vi "2 - Event vs Queue Benchmark.vi"() -> ()   [LabVIEW 2012]
uses:
  <vilib>/picture/picture.llb/imagedata.ctl
panel:
  out "Queue 2":cluster{u32, u32, u32}[](array[cluster])=[{8, 476, 0}, {8, 479, 0}, {6, 476, 0}, {7, 480, 0}, {8, 553, 0}, {8, 483, 0}, {8, 475, 0}, {9, 578, 0}, {10, 578, 0}, {8, 478, 0}, {9, 503, 0}, {9, 573, 0}, {8, 530, 0}, {8, 476, 0}, {8, 478, 0}, {8, 480, 0}, {8, 501, 0}, {7, 481, 0}, {7, 499, 0}, {7, 480, 0}]
  out "Event":cluster{u32, u32, u32}[](array[cluster])=[{24, 585, 0}, {22, 555, 0}, {21, 500, 0}, {23, 505, 0}, {25, 507, 0}, {24, 517, 0}, {20, 506, 0}, {23, 505, 0}, {23, 570, 0}, {23, 503, 0}, {23, 523, 0}, {23, 589, 0}, {25, 701, 0}, {24, 716, 0}, {25, 675, 1}, {24, 650, 0}, {22, 585, 0}, {25, 612, 0}, {22, 502, 0}, {23, 499, 0}]
  out "Time to Create":u32
  out "Time to Enqueue":u32
  out "Time to Handle":u32
  out "MB Buffered":dbl
  out "Picture 1":picture
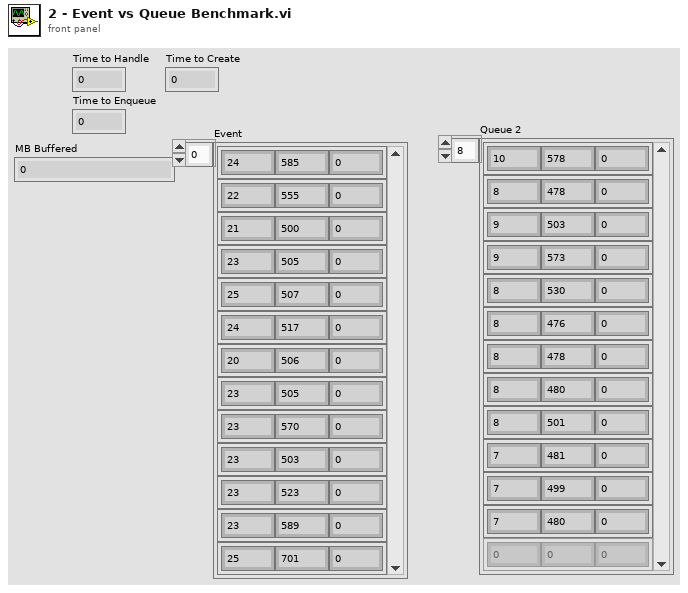
[diagram p1: front panel]
types:
  T1 = typedef "imagedata.ctl" = cluster{"image type":i32, "image depth":i32, "image":u8[], "mask":u8[], "colors":u32[], "Rectangle":cluster{"left":i16, "top":i16, "right":i16, "bottom":i16}}
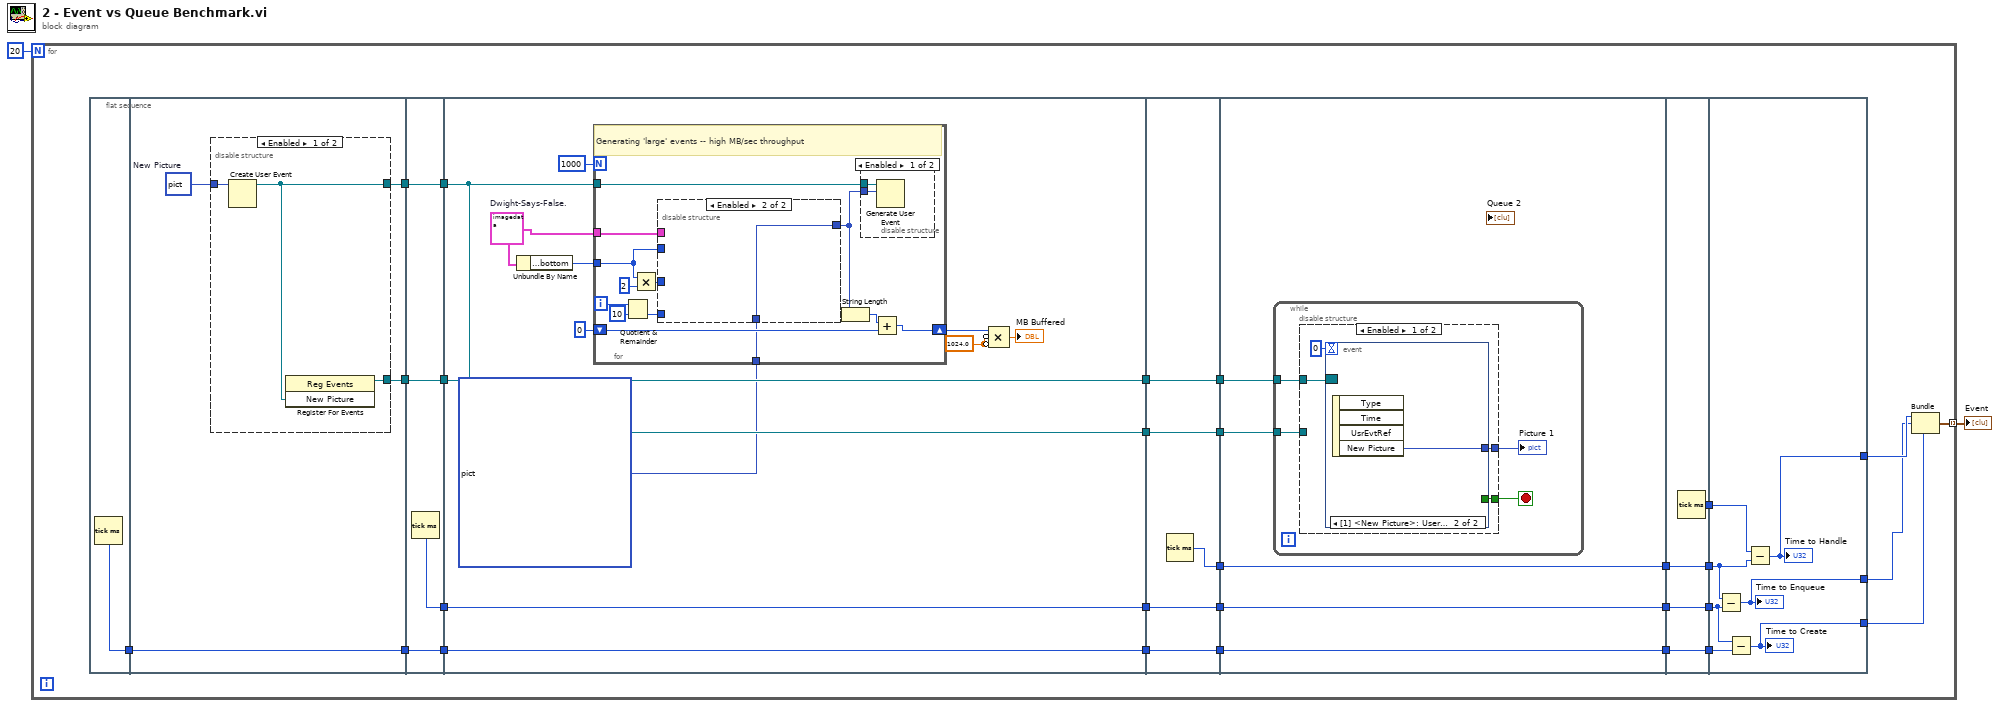
[diagram p0: block diagram]
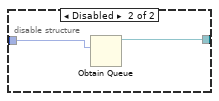
[diagram p2: hidden frame]
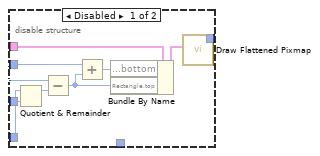
[diagram p3: hidden frame]
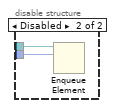
[diagram p4: hidden frame]
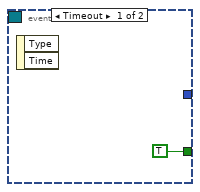
[diagram p5: hidden frame]
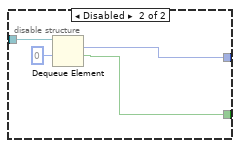
[diagram p6: hidden frame]
diagram:
  n1 = for {
    N: 20 -> [_]
    tunnel: [w3] -> w1 mode=indexing
    n2 = flat-sequence {
      tunnel: [w31] -> w30
      tunnel: [w35] -> w29
      tunnel: [w34] -> w28
      tunnel: w30 -> [w32]
      tunnel: [w32] -> w27
      tunnel: w29 -> [w44]
      tunnel: [w44] -> w26
      tunnel: w28 -> [w43]
      tunnel: [w43] -> w25
      tunnel: [w42] -> w24
      tunnel: w27 -> [w41]
      tunnel: [w41] -> w23
      tunnel: w26 -> [w49]
      tunnel: w25 -> [w50]
      tunnel: [w50] -> w22
      tunnel: [w49] -> w21
      tunnel: w24 -> [w48]
      tunnel: [w48] -> w20
      tunnel: w23 -> [w47]
      tunnel: [w47] -> w19
      tunnel: w22 -> [w88]
      tunnel: [w88] -> w18
      tunnel: [w87] -> w17
      tunnel: w21 -> [w87]
      tunnel: [w86] -> w16
      tunnel: w20 -> [w85]
      tunnel: [w85] -> w15
      tunnel: w19 -> [w84]
      tunnel: [w84] -> w14
      tunnel: w18 -> [w93]
      tunnel: w17 -> [w92]
      tunnel: [w91] -> w13
      tunnel: w16 -> [w91]
      tunnel: w15 -> [w90]
      tunnel: [w90] -> w12
      tunnel: w14 -> [w89]
      tunnel: [w89] -> w11
      tunnel: [w111] -> w10
      tunnel: [w110] -> w9
      tunnel: w13 -> [w110]
      tunnel: w12 -> [w109]
      tunnel: [w109] -> w8
      tunnel: w11 -> [w108]
      tunnel: [w108] -> w7
      tunnel: w10 -> [w118]
      tunnel: w9 -> [w117]
      tunnel: w8 -> [w116]
      tunnel: w7 -> [w115]
      tunnel: [w114] -> w6
      tunnel: [w113] -> w5
      tunnel: [w112] -> w4
      frame #0 {
        n3 = Tick Count (ms)() -> (millisecond timer value=w31:u32)
      }
      frame #1 {
        w33 = picture data[5B]  # New Picture
        n4 = disable-structure shown="Enabled" {
          disable-tunnel: [w38 w39] -> w35
          disable-tunnel: [w37 _] -> w34
          disable-tunnel: w33 -> [w36 w40]
          frame Enabled {
            n5 = Create User Event(user event datatype=w36) -> (user event=w38:refnum<user-event>)  [unwired: 1 in, 1 out]
            n6 = register-events(w38) -> (reference out=w37:refnum<event-registration>)  [unwired: 2 in, 1 out]
          }
          frame Disabled {
            n7 = Obtain Queue(element data type=w40) -> (queue out=w39:refnum<queue>)  [unwired: 4 in, 2 out]
          }
        }
      }
      frame #2 {
        n8 = Tick Count (ms)() -> (millisecond timer value=w42:u32)
      }
      frame #3 {
        w54 = 1024.0 ("value")
        w46 = T1 {"image type"=0, "image depth"=32, "image"=array[234768 elements], "mask"=array[7504 elements], "colors"=[], "Rectangle"={"left"=0, "top"=0, "right"=219, "bottom"=268}}  # Dwight-Says-False.
        n9 = Unbundle By Name(w46) -> ("Rectangle.bottom"=w51:i16)
        n10 = for {
          N: 1000 -> [_]
          tunnel: w49 -> [w69]
          tunnel: w46 -> [w68]
          tunnel: w51 -> [w62]
          shift-right: [w58] -> w55
          shift-left: 0 -> [w59]
          tunnel: picture bytes[183610] ("new picture") -> [w57]
          i -> [w65]
          # "Generating 'large' events -- high MB/sec throughput"
          n11 = Quotient & Remainder(x=w65, y=10) -> (floor(x/y)=w67:i32)  [unwired: 1 out]
          n12 = Multiply(x=w62, y=i16 2) -> (x*y=w63:i16)
          n13 = disable-structure shown="Enabled" {
            disable-tunnel: w68 -> [w77 _]
            disable-tunnel: w67 -> [w76 _]
            disable-tunnel: w63 -> [w72 _]
            disable-tunnel: w62 -> [w71 _]
            disable-tunnel: [w70 w79] -> w61
            disable-tunnel: w57 -> [_ w79]
            frame Disabled {
              n14 = Quotient & Remainder(x=w76, y=w72) -> (x-y*floor(x/y)=w74:i32)  [unwired: 1 out]
              n15 = Subtract(x=w71, y=w74) -> (x-y=w73:i32)
              n16 = Add(x=w71, y=w73) -> (x+y=w75:i32)
              n17 = Bundle By Name(cluster=w77, "Rectangle.bottom"=w75, "Rectangle.top"=w73) -> (w78:T1)
              n18 = call <vilib>:"Draw Flattened Pixmap.vi"("image data"=w78) -> ("new picture"=w70:picture)  [unwired: 8 in]
            }
            frame Enabled {
            }
          }
          n19 = String Length(string=w61) -> (length=w60:i32)
          n20 = disable-structure shown="Enabled" {
            disable-tunnel: w69 -> [w81 w83]
            disable-tunnel: w61 -> [w80 w82]
            frame Enabled {
              n21 = Generate User Event(user event=w81, event data cluster=w80) -> ()  [unwired: 1 in, 2 out]
            }
            frame Disabled {
              n22 = Enqueue Element(queue=w83, element=w82) -> ()  [unwired: 2 in, 3 out]
            }
          }
          n23 = Add(x=w60, y=w59) -> (x+y=w58:i32)
        }
        n24 = Compound Arithmetic op=MULTIPLY(w55, invert w54, invert w54) -> (→"MB Buffered":dbl)
      }
      frame #4 {
        n25 = Tick Count (ms)() -> (millisecond timer value=w86:u32)
      }
      frame #5 {
        n26 = while {
          tunnel: w93 -> [w96]
          tunnel: w92 -> [w94]
          stop <- w97 stop-if-true
          n27 = disable-structure shown="Enabled" {
            disable-tunnel: [w100 w106] -> w97
            disable-tunnel: w96 -> [w99 _]
            disable-tunnel: [w98 w104] -> w95
            disable-tunnel: w94 -> [_ w107]
            frame Enabled {
              n28 = event shown="[1] <New Picture>: User Event" {
                selector: w99 -> [_ _]
                dyn-events: _ -> [_ _]
                timeout: 0 -> [_ _]
                tunnel: [TRUE _] -> w100
                tunnel: [_ w103] -> w98
                event Timeout {
                  n29 = event-data() -> ()  [unwired: 1 in, 2 out]
                }
                event User Event {
                  n30 = event-data() -> ("New Picture"=w103:picture)  [unwired: 1 in, 3 out]
                }
              }
            }
            frame Disabled {
              n31 = Dequeue Element(queue=w107, timeout in ms (-1)=0) -> (element=w104:picture, timed out?=w106:bool)  [unwired: 1 in, 2 out]
            }
          }
          "Picture 1" <- w95
        }
      }
      frame #6 {
        n32 = Tick Count (ms)() -> (millisecond timer value=w111:u32)
      }
      frame #7 {
        n33 = Subtract(x=w117, y=w116) -> (x-y=w113:u32)
        "Time to Enqueue" <- w113
        n34 = Subtract(x=w116, y=w115) -> (x-y=w112:u32)
        "Time to Create" <- w112
        n35 = Subtract(x=w118, y=w117) -> (x-y=w114:u32)
        "Time to Handle" <- w114
      }
    }
    n36 = Bundle(w6, w5, w4) -> (w3:cluster{u32, u32, u32})  [unwired: 1 in]
  }
  "Event" <- w1
